vi "Timed Loop Test.vi"() -> ()   [LabVIEW 2026]
uses:
  <vilib>/Platform/TimedLoop/XDataNode/timing_clust.ctl
  <vilib>/Platform/TimedLoop/XDataNode/nitl_modes.ctl
  <vilib>/Platform/TimedLoop/XDataNode/wakeup.ctl
  <vilib>/platform/TimedLoop/XDataNode/XDataNode.xnode
  <vilib>/Platform/TimedLoop/XDataNode/XDNodeRunTimeDep.lvlib
panel:
  out "Numeric 2":i32
  out "Numeric":i32
  out "Loop 2":i32
  out "Loop 1":i32
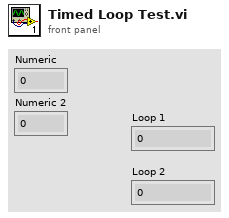
[diagram p1: front panel]
types:
  T1 = typedef "XDNodeRunTimeDep.lvlib/timing_clust.ctl" = cluster{"Expected End [f-1]":u64, "Actual End [f-1]":u64, "Finished Late? [f-1]":bool, "Expected End [i-1]":u64, "Actual End [i-1]":u64, "Finished Late? [i-1]":bool, "Expected Start [i]":u64, "Actual Start [i]":u64, "Expected Start [f]":u64, "Actual Start [f]":u64, "Source Name":string, "Structure Name":string, "Period":i64, "Deadline":i64, "Offset":i64, "Start":i64, "Priority":i32, "Timeout":i32, "Mode":T2, "Wakeup Reason":T3, "Error":errorcluster, "Source Type":string, "Secondary Source Type":string, "Global End Time":u64, "Global Start Time":u64, "Frame Duration":u64, "Iteration Duration":u64, "Assigned CPU":i32, "I/O Scan Engine Mode":u32}
  T2 = typedef "XDNodeRunTimeDep.lvlib/nitl_modes.ctl" = enum32{"No Change", "Process missed periods, maintain original phase", "Discard missed periods, maintain original phase", "Process missed periods, ignore original phase", "Discard missed periods, ignore original phase"}
  T3 = typedef "XDNodeRunTimeDep.lvlib/wakeup.ctl" = enum32{"Normal", "Aborted", "Asynchronous wakeup", "Timing source error", "Timed loop error", "Timeout"}
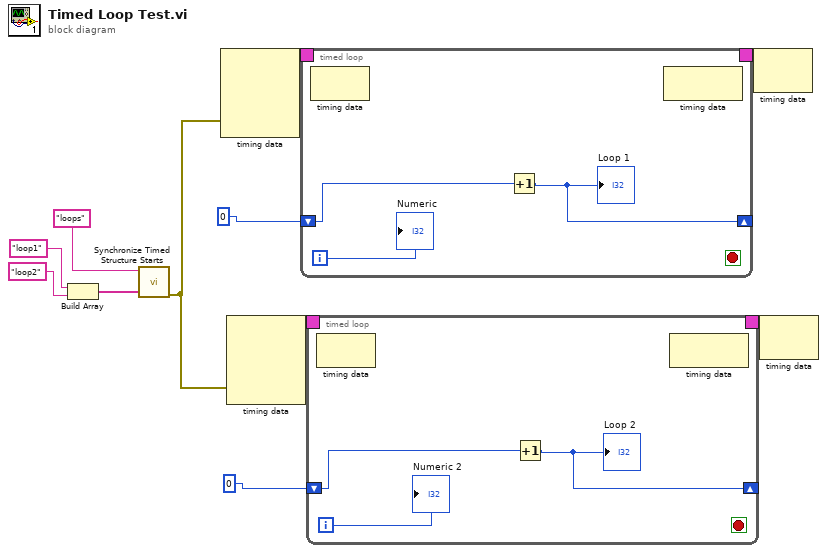
[diagram p0: block diagram]
diagram:
  n1 = Build Array("loop1", "loop2") -> (w4:string[])
  n2 = call <vilib>:"Synchronize Timed Structure Starts.vi"("timed structure names"=w4, "synchronization group name"="loops") -> ("error out"=w1:errorcluster)  [unwired: 8 in, 1 out]
  n3 = node-c288(w1) -> (w11:T1)  [unwired: 3 in]
  n4 = node-c288(w1) -> (w8:T1)  [unwired: 3 in]
  n5 = timed-loop {
    timing: w11 -> [_]
    timing-out: [_] -> w10
    shift-right: [w13] -> _
    shift-left: 0 -> [w14]
    i -> [w12]
    stop <- _ stop-if-true
    n6 = node-c288() -> ()  [unwired: 1 in, 1 out]
    n7 = Increment(x=w14) -> (x+1=w13:i32)
    "Loop 1" <- w13
    n8 = node-c288() -> ()  [unwired: 1 in, 1 out]
    "Numeric" <- w12
  }
  n9 = timed-loop {
    timing: w8 -> [_]
    timing-out: [_] -> w7
    shift-right: [w18] -> _
    shift-left: 0 -> [w19]
    i -> [w17]
    stop <- _ stop-if-true
    n10 = node-c288() -> ()  [unwired: 1 in, 1 out]
    n11 = Increment(x=w19) -> (x+1=w18:i32)
    "Loop 2" <- w18
    n12 = node-c288() -> ()  [unwired: 1 in, 1 out]
    "Numeric 2" <- w17
  }
  n13 = node-c288(w10) -> ()  [unwired: 1 out]
  n14 = node-c288(w7) -> ()  [unwired: 1 out]
